vi "Main.vi"() -> ()   [LabVIEW 2022 SP3]
uses:
  Comics/Comics.lvclass
panel:
  out "error out":errorcluster
  in  "ReadComicCache":bool
  in  "SaveComicCache":bool
  in  "GenCharList":bool
  out "Status":string
  in  "LoadComics":bool
  in  "stop":bool
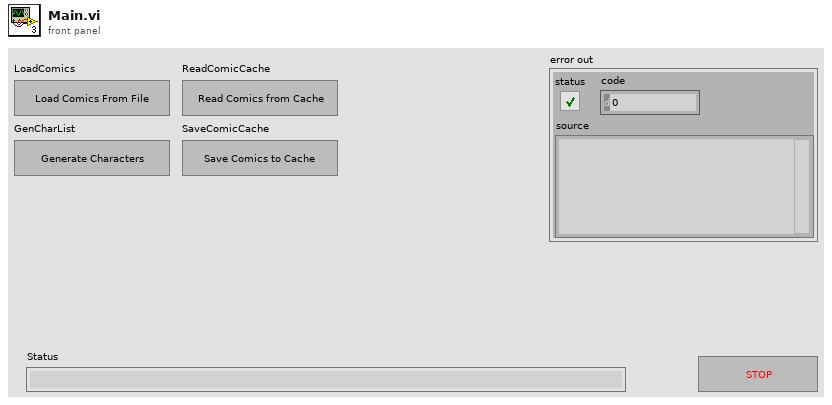
[diagram p1: front panel]
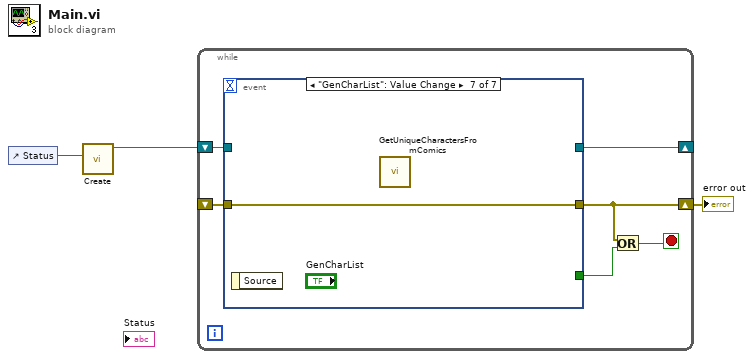
[diagram p0: block diagram]
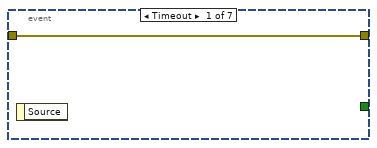
[diagram p2: hidden frame]
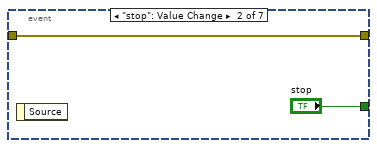
[diagram p3: hidden frame]
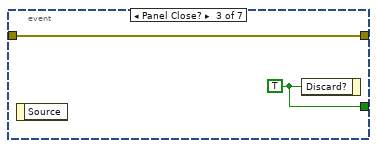
[diagram p4: hidden frame]
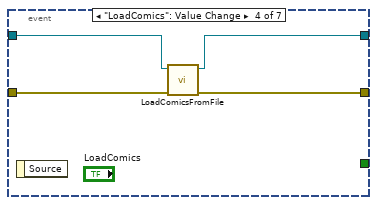
[diagram p5: hidden frame]
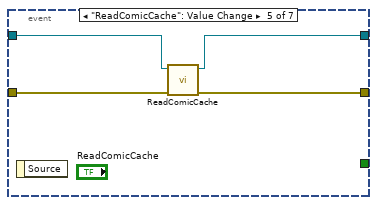
[diagram p6: hidden frame]
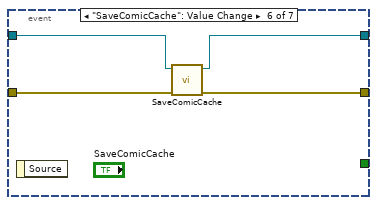
[diagram p7: hidden frame]
diagram:
  n1 = control-ref of="Status"() -> (w3:refnum<vi>)
  n2 = call "Create.vi"("Status ref"=w3) -> ("Comics.lvclass"=w2:refnum<class "Comics.lvclass">)  [unwired: 10 in]
  n3 = while {
    shift-right: [w7] -> w1
    shift-left: _ -> [w9]
    shift-right: [w4] -> _
    shift-left: w2 -> [w5]
    stop <- w8 stop-if-true
    n4 = event shown="[6] \"GenCharList\": Value Change" {
      selector: _ -> [_ _ _ _ _ _ _]
      dyn-events: _ -> [_ _ _ _ _ _ _]
      timeout: _ -> [_ _ _ _ _ _ _]
      tunnel: [_ "stop" w14 _ _ _ _] -> w6
      tunnel: [w10 w11 w13 w17 w21 w25 w27] -> w7
      tunnel: w9 -> [w10 w11 w13 w18 w22 w26 w27]
      tunnel: w5 -> [_ _ _ w16 w20 w24 _]
      tunnel: [_ _ _ w15 w19 w23 _] -> w4
      event Timeout {
        n5 = event-data() -> ()  [unwired: 1 in, 1 out]
      }
      event "stop": Value Change {
        n6 = event-data() -> ()  [unwired: 1 in, 1 out]
      }
      event Panel Close? {
        w14 = TRUE ("Discard?")
        n7 = event-data() -> ()  [unwired: 1 in, 1 out]
        n8 = event-data("Discard?"=w14) -> ()  [unwired: 1 in, 1 out]
      }
      event "LoadComics": Value Change {
        n9 = event-data() -> ()  [unwired: 1 in, 1 out]
        n10 = call "LoadComicsFromFile.vi"("error in (no error)"=w18, "Comics in"=w16) -> ("error out"=w17:errorcluster, "Comics out"=w15:refnum<class "Comics.lvclass">)  [unwired: 8 in]
      }
      event "ReadComicCache": Value Change {
        n11 = event-data() -> ()  [unwired: 1 in, 1 out]
        n12 = call "ReadComicCache.vi"("error in (no error)"=w22, "Comics in"=w20) -> ("error out"=w21:errorcluster, "Comics out"=w19:refnum<class "Comics.lvclass">)  [unwired: 8 in]
      }
      event "SaveComicCache": Value Change {
        n13 = event-data() -> ()  [unwired: 1 in, 1 out]
        n14 = call "SaveComicCache.vi"("error in (no error)"=w26, "Comics in"=w24) -> ("error out"=w25:errorcluster, "Comics out"=w23:refnum<class "Comics.lvclass">)  [unwired: 8 in]
      }
      event "GenCharList": Value Change {
        n15 = event-data() -> ()  [unwired: 1 in, 1 out]
        n16 = call "GetUniqueCharactersFromComics.vi"() -> ()  [unwired: 10 in, 2 out]
      }
    }
    n17 = Or(x=w7, y=w6) -> (x .or. y?=w8:bool)
  }
  "error out" <- w1
